vi "Init.vi"(3 "Container State":T5, 4 "Previous State":variant=variant(cluster{"Button Text":string, "Current Color":cluster{"Button":u32, "Text":u32}, "Button Color":cluster{"Button":u32, "Text":u32}, "Hover Color":cluster{"Button":u32, "Text":u32}} {"Button Text"="Test", "Current Color"={"Button"=16860, "Text"=16448250}, "Button Color"={"Button"=16860, "Text"=16448250}, "Hover Color"={"Button"=16776960, "Text"=0}}), 5 "Previous Version":T4={"Major"=1, "Minor"=0, "Fix"=0, "Build"=0}) -> (2 "Current State":T1={"On Text"="", "Off Text"="", "Current Color"={"On Color"=16860, "Text Color"=16777226, "Off Color"=16860}, "Button Color"={"On Color"=16860, "Text Color"=16777226, "Off Color"=16860}, "Hover Color"={"On Color"=16776960, "Text Color"=0, "Off Color"=16776960}, "Show Boolean Text"=TRUE, "Multiple Strings"=FALSE, "Font"={"Font Name"="", "Size"=0, "Bold"=FALSE, "Italic"=FALSE, "Underline"=FALSE, "Strikeout"=FALSE, "Alignment"=enum."Left"}})   [LabVIEW 2012, in "Hover Button.xctl"]
doc: "This Init vi gives the new instance of the hover button it's initial color properties and also remembers any saved state of each instance of the hover button when existing vis are opened that have a hover button on the front panel."
uses:
  Hover Button.xctl
  State.ctl
  Button Colors.ctl
  Font Properties.ctl
  <vilib>/_xctls/Container State.ctl
  <vilib>/_xctls/Version.ctl
  <vilib>/_xctls/XControlSupport.lvlib
panel:
  in  "Default Indicator State":T1={"On Text"="On", "Off Text"="Off", "Current Color"={"On Color"=16860, "Text Color"=16777226, "Off Color"=16860}, "Button Color"={"On Color"=16860, "Text Color"=16777226, "Off Color"=16860}, "Hover Color"={"On Color"=16776960, "Text Color"=0, "Off Color"=16776960}, "Show Boolean Text"=TRUE, "Multiple Strings"=FALSE, "Font"={"Font Name"="Arial", "Size"=18, "Bold"=TRUE, "Italic"=FALSE, "Underline"=FALSE, "Strikeout"=FALSE, "Alignment"=enum."Left"}}
  in  "Default Control State":T1={"On Text"="On", "Off Text"="Off", "Current Color"={"On Color"=16860, "Text Color"=16777226, "Off Color"=16860}, "Button Color"={"On Color"=16860, "Text Color"=16777226, "Off Color"=16860}, "Hover Color"={"On Color"=16776960, "Text Color"=0, "Off Color"=16776960}, "Show Boolean Text"=TRUE, "Multiple Strings"=FALSE, "Font"={"Font Name"="Arial", "Size"=18, "Bold"=TRUE, "Italic"=FALSE, "Underline"=FALSE, "Strikeout"=FALSE, "Alignment"=enum."Left"}}
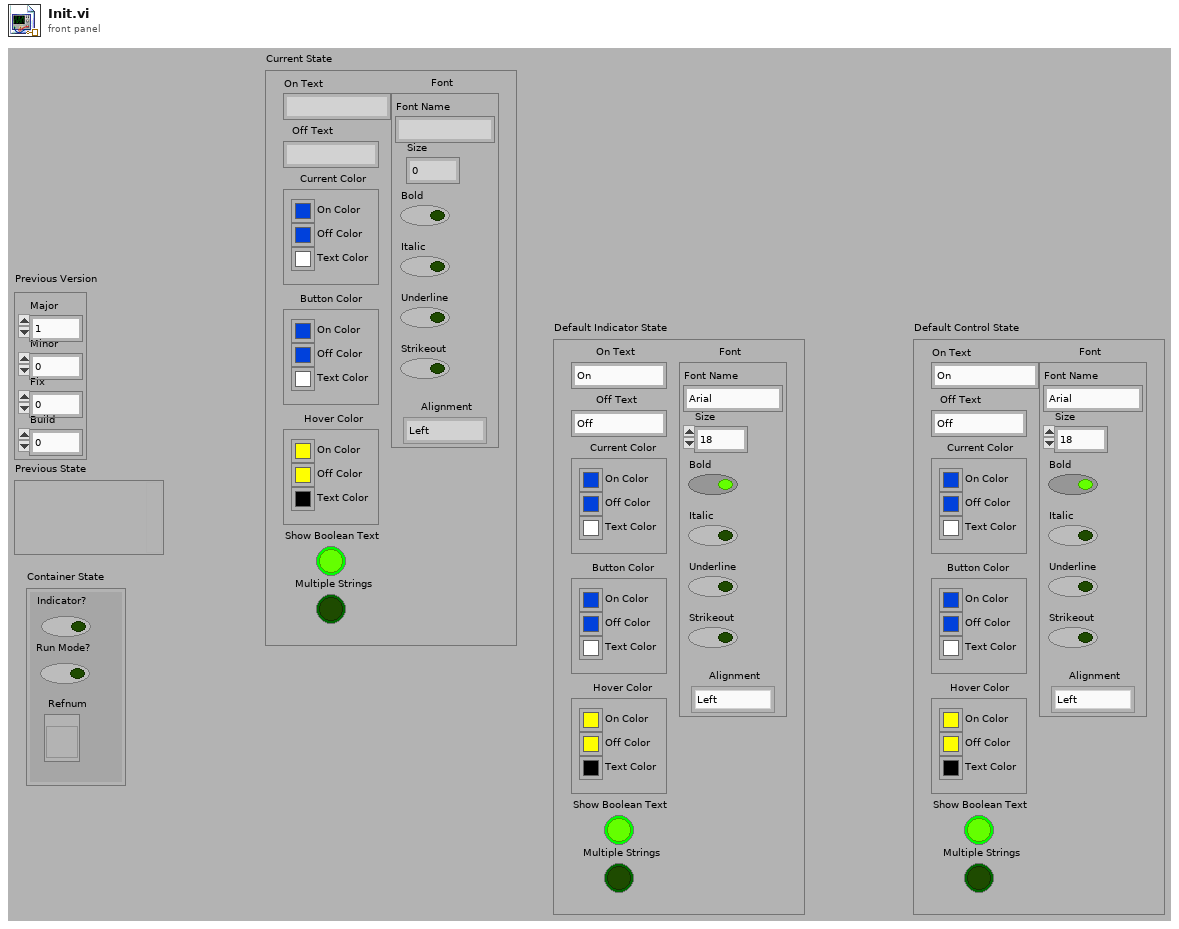
[diagram p1: front panel]
types:
  T1 = typedef "Hover Button.xctl/State.ctl" = cluster{"On Text":string, "Off Text":string, "Current Color":T2, "Button Color":T2, "Hover Color":T2, "Show Boolean Text":bool, "Multiple Strings":bool, "Font":T3}
  T2 = typedef "Hover Button.xctl/Button Colors.ctl" = cluster{"On Color":u32, "Text Color":u32, "Off Color":u32}
  T3 = typedef "Hover Button.xctl/Font Properties.ctl" = cluster{"Font Name":string, "Size":u32, "Bold":bool, "Italic":bool, "Underline":bool, "Strikeout":bool, "Alignment":enum16{"Left", "Center", "Right"}}
  T4 = typedef "XControlSupport.lvlib/Version.ctl" = cluster{"Major":u16, "Minor":u16, "Fix":u16, "Build":u16}
  T5 = typedef "XControlSupport.lvlib/Container State.ctl" = cluster{"Indicator?":bool, "Run Mode?":bool, " Refnum":refnum<vi>}
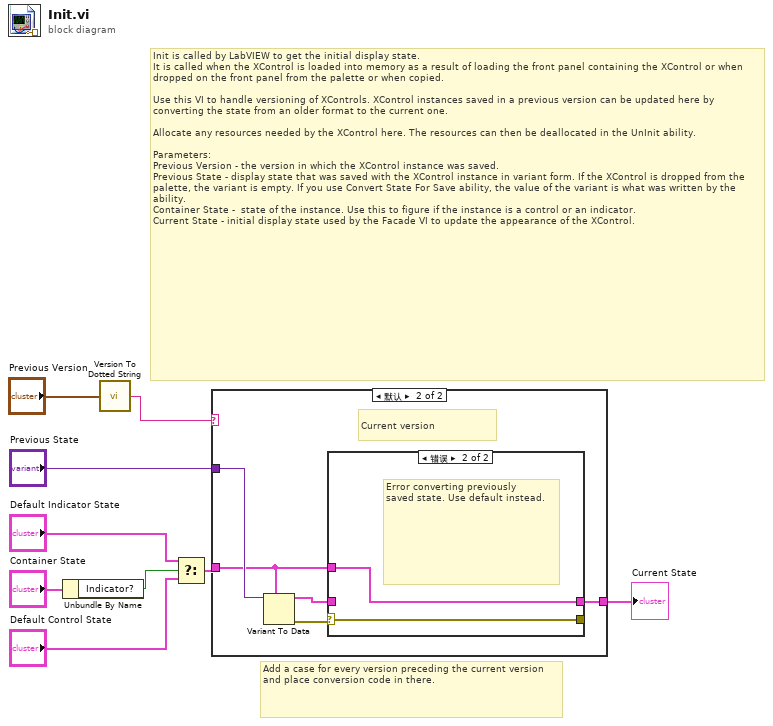
[diagram p0: block diagram]
diagram:
  # "Add a case for every version preceding the current version and place conversion code in there."
  # "Init is called by LabVIEW to get the initial display state.\nIt is called when the XControl is loaded into memory as a result of loading the front panel containing the XControl or when dropped on the front panel from the palette or when copied.\n\nUse this VI to handle versioning of XControls. XControl instances saved in a previous version can be updated here by converting the state from an older format to the current one.\n\nAllocate any resources needed by the XControl here. The resources can then be deallocated in the UnInit ability.\n\nParameters:\nPrevious Version - the version in which the XControl instance was saved.\nPrevious State - display state that was saved with the XControl instance in variant form. If the XControl is dropped from the palette, the variant is empty. If you use Convert State For Save ability, the value of the variant is what was written by the ability. \nContainer State -  state of the instance. Use this to figure if the instance is a control or an indicator.\nCurrent State - initial display state used by the Facade VI to update the appearance of the XControl."
  n1 = Unbundle By Name("Container State") -> ("Indicator?"=w4:bool)
  n2 = call <vilib>:"Version To Dotted String.vi"("Version"="Previous Version") -> ("String Version"=w1:string)
  n3 = Select(t="Default Indicator State", s=w4, f="Default Control State") -> (s? t:f=w3:T1)
  n4 = case shown="默认" w1 {
    tunnel: "Previous State" -> [_ w15]
    tunnel: [w10 w11] -> w8
    tunnel: w3 -> [w10 w12]
    frame "0.0.0.0" {
      # "Just created, use default state"
    }
    frame Default {
      # "Current version"
      n5 = Variant To Data(type=w12, Variant=w15) -> (data=w13:T1, error out=w14:errorcluster)  [unwired: 1 in]
      n6 = case shown="错误" w14 {
        selector: w14 -> [w17 w18]
        tunnel: w13 -> [w16 _]
        tunnel: [w16 w19] -> w11
        tunnel: w12 -> [_ w19]
        tunnel: [w17 w18] -> _
        frame No Error {
        }
        frame Error {
          # "Error converting previously \nsaved state. Use default instead."
        }
      }
    }
  }
  "Current State" <- w8
